vi "IterateDrive.vi"   [LabVIEW 2015]
doc: "Drive will iterate through the given values and access the speed as well.\n The difference in the speed will be accessed from left joystick engaging for fire."
uses:
  <vilib>/Rock Robotics/WPI/Utilities/WPI_GetSetVariantRefNum.vi
  <vilib>/Rock Robotics/Network Tables/NT Write Numeric Array.vi
types:
  T1 = typedef "WPI_JoystickDevRef.ctl" = cluster{"Device":T2}
  T2 = typedef "WPI_JoystickDeviceEnum.ctl" = enum16{"USB 0", "USB 1", "USB 2", "USB 3", "USB 4", "USB 5"}
  T3 = typedef "WPI_RobotDriveDevRef.ctl" = cluster{"DevStatus":errorcluster, "Motors[]":T4[], "Square Inputs":bool, "Max Output":dbl}
  T4 = typedef "WPI_MotorControlDeviceRef.ctl" = cluster{"DeviceStatus":errorcluster, "Type":T5, "PWM":cluster{"PWM Channel":T6, "DeadBand":T7}, "CAN":cluster{"Device Number":u8, "Control Mode":T8, "Semaphore":T9, "Max Vout":dbl, "TalonSRX Control Mode":T10}, "Invert":bool}
  T5 = typedef "WPI_MotorControlType.ctl" = enum16{"PWM", "CAN", "CANTalonSRX"}
  T6 = typedef "FPGA_DIOPWMChannel.ctl" = enum8{"PWM 0", "PWM 1", "PWM 2", "PWM 3", "PWM 4", "PWM 5", "PWM 6", "PWM 7", "PWM 8", "PWM 9", "PWM MXP 0", "PWM MXP 1", "PWM MXP 2", "PWM MXP 3", "PWM MXP 4", "PWM MXP 5", "PWM MXP 6", "PWM MXP 7", "PWM MXP 8", "PWM MXP 9", "Invalid"}
  T7 = typedef "WPI_PWMDeadband.ctl" = cluster{"Name":string, "maxPositivePwm":i32, "minPositivePwm":i32, "centerPwm":i32, "maxNegativePwm":i32, "minNegativePwm":i32, "angularRange":u16}
  T8 = typedef "WPI_CANJaguar_ControlMode.ctl" = enum8{"Percent VBus", "Current", "Speed", "Position", "Voltage"}
  T9 = typedef "Semaphore RefNum" = refnum<k1>
  T10 = typedef "WPI_CANTalonSRX_APIControlMode.ctl" = enum8{"Percent VBus", "Speed", "Position", "Slave", "Unchanged / Invalid", "Voltage Compensation", "Current", "Motion Profile"}
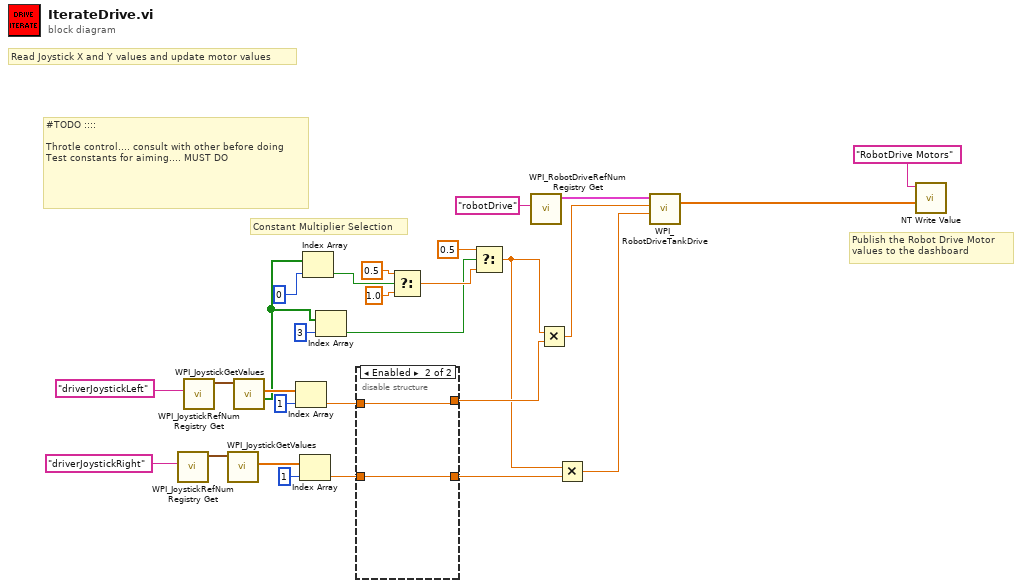
[diagram p0: block diagram]
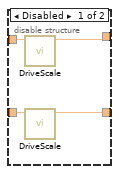
[diagram p2: hidden frame]
diagram:
  # "#TODO :::: \n\nThrotle control.... consult with other before doing\nTest constants for aiming.... MUST DO"
  # "Constant Multiplier Selection"
  # "Publish the Robot Drive Motor\nvalues to the dashboard"
  # "Read Joystick X and Y values and update motor values"
  n1 = call <vilib>:"WPI_JoystickRefNum Registry Get.vi"("refnum name"="driverJoystickRight") -> ("JoystickDevRef"=w27:T1)  [unwired: 1 in, 9 out]
  n2 = call <vilib>:"WPI_JoystickRefNum Registry Get.vi"("refnum name"="driverJoystickLeft") -> ("JoystickDevRef"=w22:T1)  [unwired: 1 in, 9 out]
  n3 = call <vilib>:"WPI_JoystickGetValues.vi"("JoystickDevRef"=w27) -> ("Axes"=w28:dbl[])  [unwired: 6 in, 4 out]
  n4 = call <vilib>:"WPI_JoystickGetValues.vi"("JoystickDevRef"=w22) -> ("Buttons"=w3:bool[], "Axes"=w23:dbl[])  [unwired: 6 in, 3 out]
  n5 = Index Array(array=w23, index=1) -> (element=w11:dbl)
  n6 = Index Array(array=w28, index=1) -> (element=w10:dbl)
  n7 = Index Array(array=w3, index=0) -> (element=w17:bool)
  n8 = Index Array(array=w3, index=3) -> (element=w1:bool)
  n9 = disable-structure shown="Enabled" {
    disable-tunnel: [w32 w34] -> w12
    disable-tunnel: w11 -> [w31 w34]
    disable-tunnel: w10 -> [w30 w33]
    disable-tunnel: [w29 w33] -> w9
    frame Disabled {
      n10 = call "DriveScale.vi"("Numeric in"=w31) -> ("Numeric out"=w32:dbl)  [unwired: 10 in]
      n11 = call "DriveScale.vi"("Numeric in"=w30) -> ("Numeric out"=w29:dbl)  [unwired: 10 in]
    }
    frame Enabled {
    }
  }
  n12 = Select(t=0.5, s=w17, f=1.0) -> (s? t:f=w6:dbl)
  n13 = Select(t=0.5, s=w1, f=w6) -> (s? t:f=w5:dbl)
  n14 = call <vilib>:"WPI_RobotDriveRefNum Registry Get.vi"("refnum name"="robotDrive") -> ("RobotDriveDevRef"=w20:T3)  [unwired: 1 in, 9 out]
  n15 = Multiply(x=w5, y=w12) -> (x*y=w14:dbl)
  n16 = Multiply(x=w5, y=w9) -> (x*y=w13:dbl)
  n17 = call <vilib>:"WPI_RobotDriveTankDrive.vi"("Right axis value"=w13, "Left axis value"=w14, "RobotDriveDevRef"=w20) -> ("Motor Values"=w24:dbl[])  [unwired: 6 in, 2 out]
  n18 = call-poly <vilib>:"NT Write Value.vi"("Numeric Array"=w24, "Name"="RobotDrive Motors") -> ()  [unwired: 9 in, 1 out]
